vi "Log Built Version.vi"(8 "error in (no error)":errorcluster, 10 "Generated PPL":path, 11 "Builder in":refnum<class "Builder.lvclass">) -> (0 "error out":errorcluster, 1 "Library Description":string, 3 "Builder out":refnum<class "Builder.lvclass">)   [LabVIEW 2019, in "Builder.lvclass"]
uses:
  Builder.lvclass
  Builder.lvclass/Builder.ctl
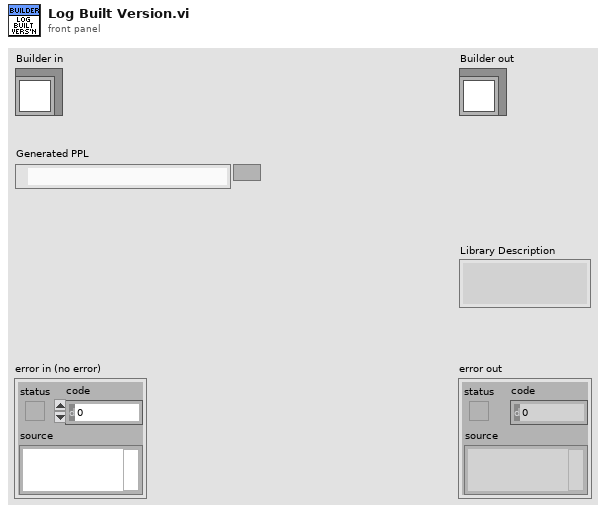
[diagram p1: front panel]
types:
  T1 = enum16{"open", "replace", "create", "open or create", "replace or create", "replace or create with confirmation"}
  T2 = cluster{"Major":i32, "Minor":i32, "Patch":i32, "Build":i32}
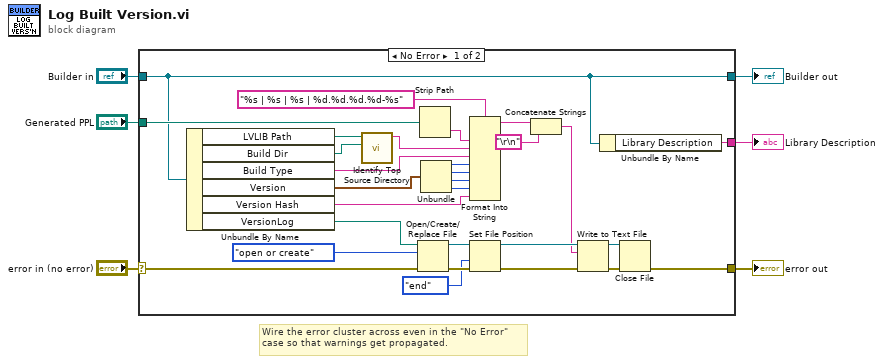
[diagram p0: block diagram]
diagram:
  # "Wire the error cluster across even in the \"No Error\"\ncase so that warnings get propagated."
  n1 = case shown="No Error" "error in (no error)" {
    selector: "error in (no error)" -> [w27 w37]
    tunnel: [w26 w37] -> w5
    tunnel: [w8 w36] -> w3
    tunnel: "Builder in" -> [w8 w36]
    tunnel: "Generated PPL" -> [w24 _]
    tunnel: [w7 _] -> w1
    frame No Error {
      n2 = Unbundle By Name(w8) -> ("LVLIB Path"=w9:path, "Build Dir"=w10:path, "Build Type"=w15:string, "Version"=w16:T2, "Version Hash"=w18:string, "VersionLog"=w14:path)
      n3 = call "Identify Top Source Directory.vi"("Build Directory"=w10, "Library Path"=w9) -> ("Library Top-Level Path"=w11:string)  [unwired: 8 in, 1 out]
      n4 = Open/Create/Replace File(file path (use dialog)=w14, error in=w27, operation (0:open)=T1."open or create") -> (refnum out=w34:refnum<file>, error out=w33:errorcluster)  [unwired: 3 in, 1 out]
      n5 = Strip Path(path=w24) -> (name=w23:string)  [unwired: 1 out]
      n6 = Unbundle(w16) -> ("Major"=w22:i32, "Minor"=w21:i32, "Patch"=w20:i32, "Build"=w19:i32)
      n7 = Format Into String(format string="%s | %s | %s | %d.%d.%d.%d-%s", w23, w11, w15, w22, w21, w20, w19, w18) -> (resulting string=w25:string)  [unwired: 2 in, 1 out]
      n8 = Set File Position(refnum=w34, from (0:start)=enum16{"start", "end", "current"}."end", error in=w33) -> (refnum out=w31:refnum<file>, error out=w30:errorcluster)  [unwired: 1 in]
      n9 = Concatenate Strings(w25, "\r\n") -> (w13:string)
      n10 = Write to Text File(file (use dialog)=w31, text=w13, error in=w30) -> (refnum out=w29:refnum<file>, error out=w28:errorcluster)  [unwired: 1 in, 1 out]
      n11 = Unbundle By Name(w8) -> ("Library Description"=w7:string)
      n12 = Close File(refnum=w29, error in=w28) -> (error out=w26:errorcluster)  [unwired: 1 out]
    }
    frame Error {
    }
  }
  "error out" <- w5
  "Builder out" <- w3
  "Library Description" <- w1
